vi "ke2002_display_value.vi"(8 "error in":errorcluster, 9 "status code":i32, 10 "temp [deg C]":dbl, 11 "VISA in":refnum<visa-resource-name>) -> (0 "error out":errorcluster, 3 "VISA out":refnum<visa-resource-name>)   [LabVIEW 2020]
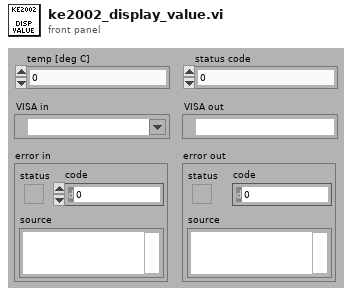
[diagram p1: front panel]
types:
  T1 = cluster{"error":bool, "code":i32, "source":string}
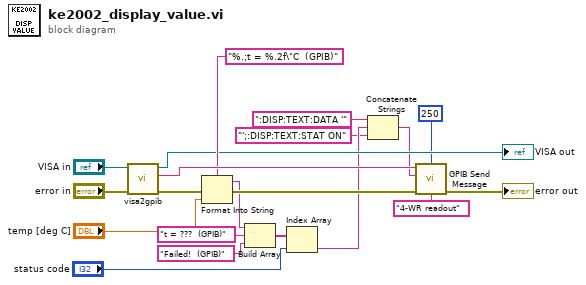
[diagram p0: block diagram]
diagram:
  n1 = call "visa2gpib.vi"("error in"="error in", "VISA in"="VISA in") -> ("error out"=w16:errorcluster, "combined address"=w15:string, "VISA out"=→"VISA out":refnum<visa-resource-name>)  [unwired: 7 in]
  n2 = Format Into String(format string="%.;t = %.2f\"C  (GPIB)", error in=w16, "temp [deg C]") -> (resulting string=w10:string, error out=w20:errorcluster)  [unwired: 1 in]
  n3 = Build Array(w10, "t = ???  (GPIB)" ("element"), "Failed!  (GPIB)" ("element")) -> (w7:string[])
  n4 = Index Array(array=w7, index="status code") -> (element=w4:string)
  n5 = Concatenate Strings(":DISP:TEXT:DATA '" ("string"), w4, "';:DISP:TEXT:STAT ON" ("string")) -> (w5:string)
  n6 = call "GPIB Send Message.vi"("timeout ms"=u32 250, "address string"=w15, "write buffer"=w5, "source"="4-WR readout", "error in"=w20) -> ("error out"=→"error out":T1)  [unwired: 2 in, 2 out]
